vi "DescribeColumns.vi"() -> ()   [LabVIEW 2014]
panel:
  out "Columns":cluster{"Columns":u16[]}[](array[cluster])
  out "Rows":i32[](array[numeric])=[0, 0, 0, 0, 0, 4]
  out "Array":string[][](array[string])=[["", "", "", "", "", "", ""], ["", "", "", "", "", "", ""], ["", "", "", "", "", "", ""], ["", "", "", "", "", "", ""], ["", "", "", "", "", "", ""], ["", "", "", "", "e6", "", "g6"]]
  in  "Table Control":string[][](table)=[["", "", "", "", "", "", ""], ["", "", "", "", "", "", ""], ["", "", "", "", "", "", ""], ["", "", "", "", "", "", ""], ["", "", "", "", "", "", ""], ["", "", "", "", "e6", "", "g6"]]
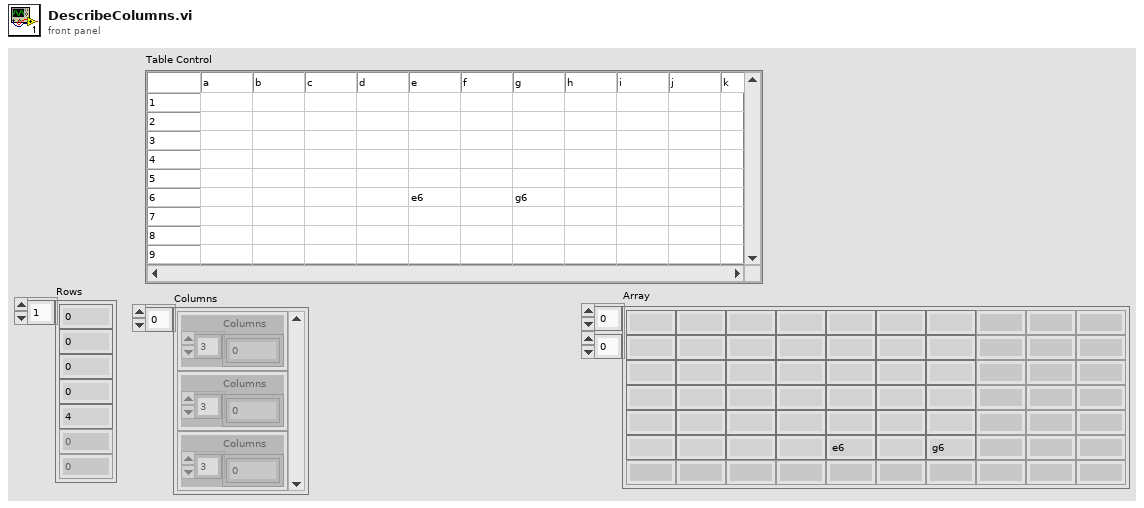
[diagram p1: front panel]
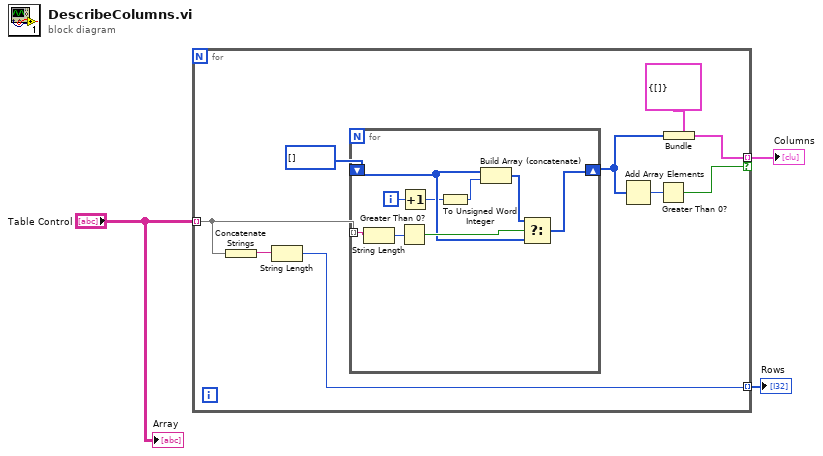
[diagram p0: block diagram]
diagram:
  n1 = for {
    tunnel: "Table Control" -> [w12] mode=indexing
    tunnel: [w10] -> w2 mode=indexing
    tunnel: [w4] -> w1 mode=indexing if=w7
    n2 = Concatenate Strings(w12) -> (w11:string)
    n3 = String Length(string=w11) -> (length=w10:i32)
    n4 = for {
      tunnel: w12 -> [w21] mode=indexing
      shift-right: [w16] -> w5
      shift-left: u16[] [] -> [w15]
      i -> [w18]
      n5 = String Length(string=w21) -> (length=w20:i32)
      n6 = Greater Than 0?(x=w20) -> (x > 0?=w19:bool)
      n7 = Increment(x=w18) -> (x+1=w14:i32)
      n8 = To Unsigned Word Integer(number=w14) -> (unsigned 16bit integer=w13:u16)
      n9 = Build Array (concatenate)(w15, w13) -> (w17:u16[])
      n10 = Select(t=w17, s=w19, f=w15) -> (s? t:f=w16:u16[])
    }
    n11 = Add Array Elements(numeric array=w5) -> (sum=w8:u16)
    n12 = Greater Than 0?(x=w8) -> (x > 0?=w7:bool)
    n13 = Bundle(cluster=cluster{"Columns":u16[]} {"Columns"=[]} ("Column"), "Columns"=w5) -> (w4:cluster{"Columns":u16[]})
  }
  "Rows" <- w2
  "Columns" <- w1
  "Array" <- "Table Control"
